vi "Read FolderName to Decrypt.vi"(8 "error in (no error)":errorcluster, 11 "Crypter in":refnum<class "Crypter.lvclass">) -> (0 "error out":errorcluster, 2 "FolderName to Decrypt":path, 3 "Crypter out":refnum<class "Crypter.lvclass">)   [LabVIEW 2016, in "Crypter.lvclass"]
uses:
  Crypter.lvclass
  Crypter.lvclass/Crypter.ctl
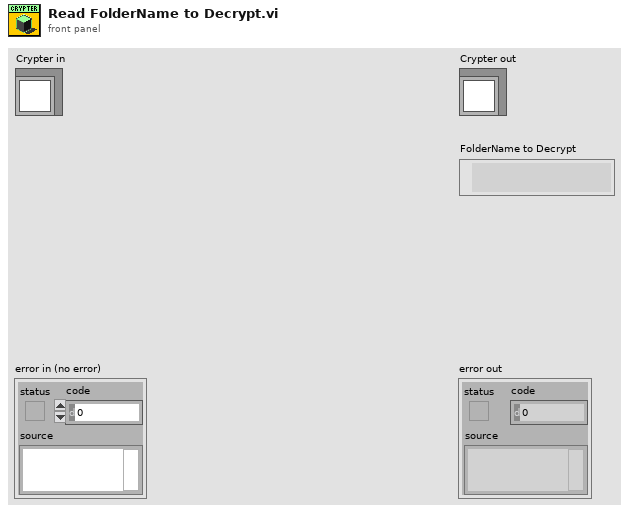
[diagram p1: front panel]
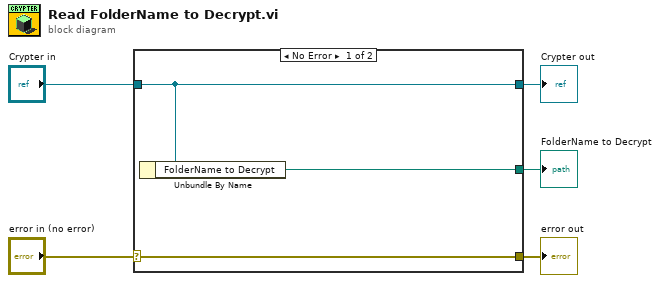
[diagram p0: block diagram]
diagram:
  n1 = case shown="No Error" "error in (no error)" {
    selector: "error in (no error)" -> [w8 w9]
    tunnel: [w8 w9] -> w4
    tunnel: [w7 w10] -> w2
    tunnel: "Crypter in" -> [w7 w10]
    tunnel: [w6 _] -> w1
    frame No Error {
      n2 = Unbundle By Name(w7) -> ("FolderName to Decrypt"=w6:path)
    }
    frame Error {
    }
  }
  "error out" <- w4
  "Crypter out" <- w2
  "FolderName to Decrypt" <- w1
